vi "sortChannels.vi"(8 "error in (no error)":errorcluster, 9 "calibratedValues":dbl[](array[numeric]), 10 "channel_addresses":string[](array[string]), 11 "DIO64Output in":refnum<class "DIO64Output.lvclass">) -> (0 "error out":errorcluster, 1 "sorted Data":dbl[](array[numeric]), 2 "sorted channels addresses":string[](array[string]), 3 "DIO64Output out":refnum<class "DIO64Output.lvclass">)   [LabVIEW 2011, in "Hardware.lvlib" / "Channels.lvlib" / "DIO64Output.lvclass"]
uses:
  DIO64Output.lvclass
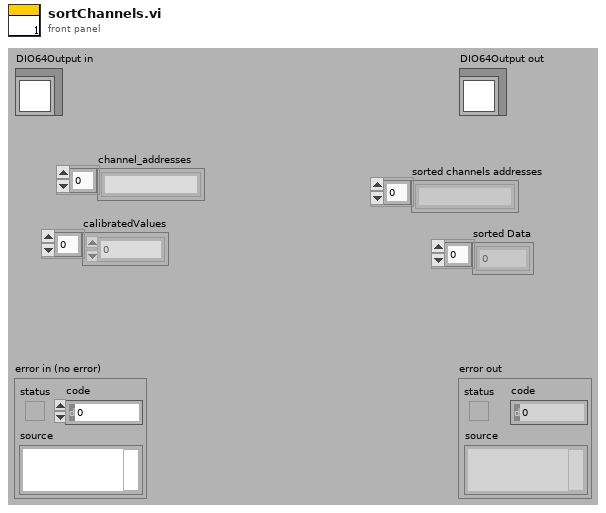
[diagram p1: front panel]
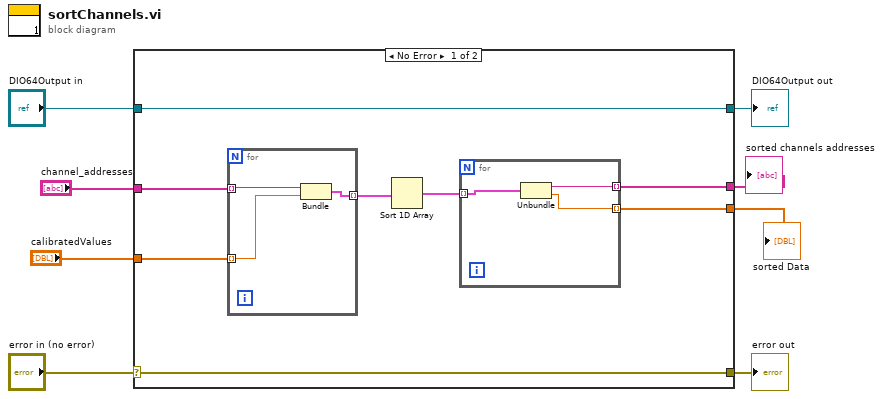
[diagram p0: block diagram]
diagram:
  n1 = case shown="No Error" "error in (no error)" {
    selector: "error in (no error)" -> [w15 w24]
    tunnel: [w15 w24] -> w7
    tunnel: [w16 w23] -> w5
    tunnel: "DIO64Output in" -> [w16 w23]
    tunnel: "channel_addresses" -> [w10 _]
    tunnel: "calibratedValues" -> [w9 _]
    tunnel: [w12 _] -> w2
    tunnel: [w11 _] -> w1
    frame No Error {
      n2 = for {
        tunnel: w10 -> [w22] mode=indexing
        tunnel: w9 -> [w21] mode=indexing
        tunnel: [w20] -> w14 mode=indexing
        n3 = Bundle(w22, "calibratedValue"=w21) -> (w20:cluster{string, "calibratedValue":dbl})  [unwired: 1 in]
      }
      n4 = Sort 1D Array(array=w14) -> (sorted array=w13:cluster{string, "calibratedValue":dbl}[])
      n5 = for {
        tunnel: w13 -> [w19] mode=indexing
        tunnel: [w18] -> w12 mode=indexing
        tunnel: [w17] -> w11 mode=indexing
        n6 = Unbundle(w19) -> (w18:string, "calibratedValue"=w17:dbl)
      }
    }
    frame Error {
    }
  }
  "error out" <- w7
  "DIO64Output out" <- w5
  "sorted channels addresses" <- w2
  "sorted Data" <- w1
